vi "Send Start Recording.vi"(7 "Message Priority (Normal)":T3=enum."Normal", 8 "error in (no error)":errorcluster, 10 "Movie Series":T2={"Camera Settings"={"Exposure Time (ms)"=100.0, "Binning"=enum."2x2", "Scan Mode"=0, "Frames to Acquire"=1000.0, "Pixel Correction"=FALSE, "Frames to Skip"=0, "File Path"=path "", "Duty cycle"=0.0, "ALEX"=FALSE, "Shutter Enable"=[], "Timelapse Interval (s)"=0}, "Auto-Advance"=TRUE, "Auto Focus"=TRUE, "Injection Countdown"=TRUE, "Movies to acquire"=1} {"Camera Settings"."Timelapse Interval (s)" max=60000 step=1; "Camera Settings"."Exposure Time (ms)" min=1.0 max=10000.0 step=1.0}, 11 "Message Enqueuer":refnum<class "Message Enqueuer.lvclass">) -> (0 "error out":errorcluster, 3 "Message Enqueuer out":refnum<class "Message Enqueuer.lvclass">)   [LabVIEW 2018, in "Application.lvlib" / "Start Recording Msg.lvclass"]
doc: "This VI sends the message to an actor."
uses:
  Start Recording Msg.lvclass
  <vilib>/ActorFramework/Message Enqueuer/Message Enqueuer.lvclass
  <vilib>/ActorFramework/Message Enqueuer/Message Priority.ctl
  Resources/Type Defs/Camera Settings.ctl
  C:/Program Files/National Instruments/LabVIEW 2018/vi.lib/ActorFramework/Message/Message.lvclass
  Start Recording Msg.lvclass/Start Recording Msg.ctl
  <vilib>/ActorFramework/Message Enqueuer/Message Enqueuer.lvclass/Message Enqueuer.ctl
  <vilib>/ActorFramework/Message Priority Queue/Priority Enqueue.vi
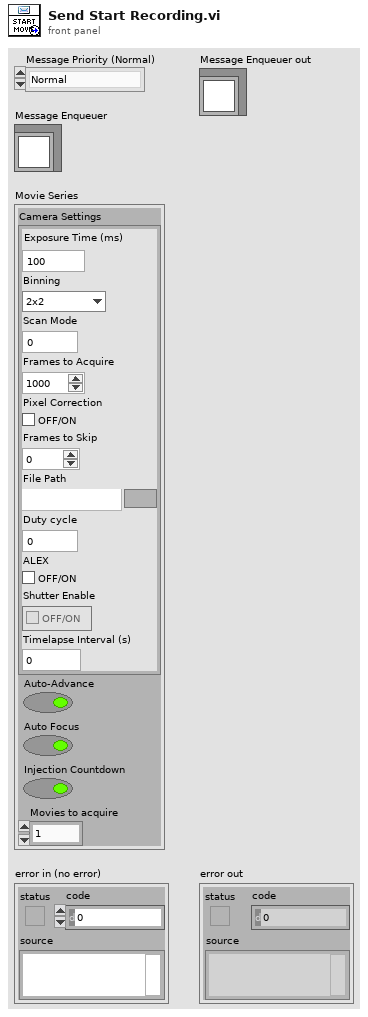
[diagram p1: front panel]
types:
  T1 = typedef "Camera Settings.ctl" = cluster{"Exposure Time (ms)":dbl, "Binning":enum16{"1x1", "2x2", "4x4"}, "Scan Mode":i32, "Frames to Acquire":dbl, "Pixel Correction":bool, "Frames to Skip":u32, "File Path":path, "Duty cycle":dbl, "ALEX":bool, "Shutter Enable":bool[], "Timelapse Interval (s)":u32}
  T2 = cluster{"Camera Settings":T1, "Auto-Advance":bool, "Auto Focus":bool, "Injection Countdown":bool, "Movies to acquire":i32}
  T3 = typedef "Actor Framework.lvlib/Message Enqueuer.lvclass/Message Priority.ctl" = enum16{"Low", "Normal", "High"}
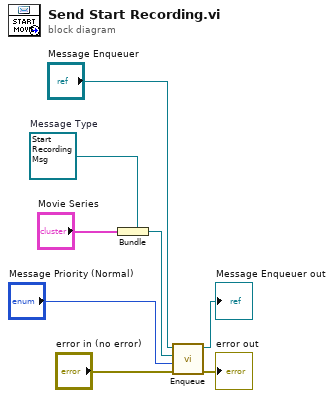
[diagram p0: block diagram]
diagram:
  w5 = refnum<class "Start Recording Msg.lvclass"> refnum  # Message Type
  n1 = Bundle(cluster=w5, "Movie Series") -> (w4:refnum<class "Start Recording Msg.lvclass">)
  n2 = call <vilib>:"Enqueue.vi"("error in (no error)"="error in (no error)", "Message Priority (Normal)"="Message Priority (Normal)", "Message"=w4, "Message Enqueuer in"="Message Enqueuer") -> ("error out"=→"error out":errorcluster, "Message Enqueuer out"=→"Message Enqueuer out":refnum<class "Message Enqueuer.lvclass">)  [unwired: 6 in]
